vi "ReadEmptyString.vi"(8 "error in (no error)":errorcluster, 11 "XuLyDataDisplay in":refnum<class "XuLyDataDisplay.lvclass">) -> (0 "error out":errorcluster, 1 "Boolean":bool, 2 "String":string, 3 "XuLyDataDisplay out":refnum<class "XuLyDataDisplay.lvclass">)   [LabVIEW 2017, in "LibraryGcode.lvlib" / "XuLyDataDisplay.lvclass"]
uses:
  XuLyDataDisplay.lvclass
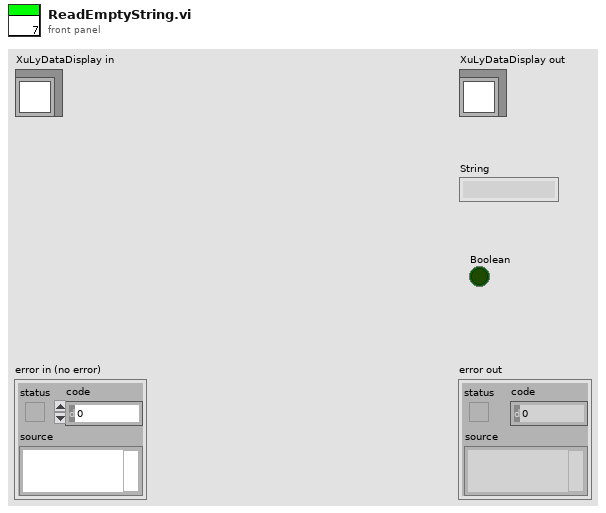
[diagram p1: front panel]
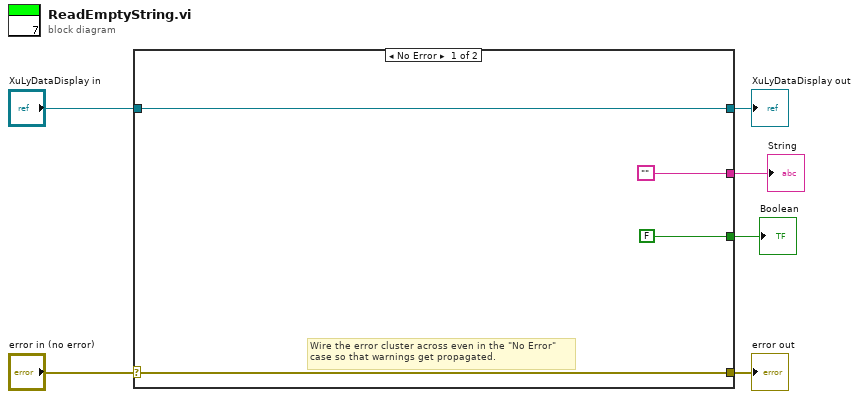
[diagram p0: block diagram]
diagram:
  n1 = case shown="No Error" "error in (no error)" {
    selector: "error in (no error)" -> [w9 w12]
    tunnel: [w9 w12] -> w5
    tunnel: [w10 w11] -> w3
    tunnel: "XuLyDataDisplay in" -> [w10 w11]
    tunnel: ["" _] -> w2
    tunnel: [FALSE _] -> w1
    frame No Error {
      # "Wire the error cluster across even in the \"No Error\"\ncase so that warnings get propagated."
    }
    frame Error {
    }
  }
  "error out" <- w5
  "XuLyDataDisplay out" <- w3
  "String" <- w2
  "Boolean" <- w1
